vi "direct_ads_vol_T_pwpsatRho.vi"(5 "Density of adsorpt in kg/m3 (Input)":dbl, 7 "Saturation pressure in Pa (Input)":dbl, 8 "Error (Input)":errorcluster, 9 "Loading in kg/kg (Input)":dbl, 10 "Pressure in Pa (Input)":dbl, 11 "WorkingPair (Input)":T1={"no_iso"=1, "no_p_sat"=1, "path_db"="D:\\Driesel\\SorpLibLocal\\LabVIEW_wrapper\\data\\json\\sorpproplib_minimalExample.json", "wp_as"="silicagel", "wp_st"="123", "wp_iso"="DubininArctan1", "wp_rf"="water", "rf_rhol"="SaturatedLiquidDensity_EoS1", "no_rhol"=1, "rf_psat"="VaporPressure_EoS1"}) -> (0 "Error (Output)":errorcluster caption="Error(Output)", 3 "Equilibrium temperature in K (Output)":dbl)   [LabVIEW 2017]
doc: "direct_ads_vol_T_pwpsatRho:\n * ---------------------------\n *\n * Calculates equilibrium temperature T in K depending on equilibrium pressure\n * in Pa, equilibrium loading w in kg/kg, saturation pressure p_Sat in Pa and\n * density of adsorpt rho in kg/m³.\n *\n * Parameters:\n * -----------\n * double p_Pa:\n * Equilibrium pressure in Pa.\n * double w_kgkg:\n * Equilibrium loading in kg/kg.\n * double p_sat_Pa:\n * Saturation pressure in Pa.\n * double rho_kgm3:\n * Density of adsorpt in kg/m³.\n *\n * const char *path_db:\n * Path to database.\n * const char *wp_as:\n * Name of sorbent.\n * const char *wp_st:\n * Name of sub-type of sorbent.\n * const char *wp_rf:\n * Name of refrigerant.\n * const char *wp_iso:\n * Name of isotherm.\n * int no_iso:\n * ID of isotherm (i.e. when more than one isotherm is available)\n * const char *rf_psat:\n * Name of calculation approach for vapor pressure.\n * int no_p_sat:\n * ID of vapor pressure equation (i.e. when more than one equation is\n * available)\n * const char *rf_rhol:\n * Name of calculation approach for liquid density.\n * int no_rhol:\n * ID of liquid density equation (i.e. when more than one equation is\n * available)\n *\n * Returns:\n * --------\n * double:\n * Equilibrium temperature in K.\n *\n * Remarks:\n * --------\n * This function is only valid for isotherm models based on the volumetric\n * approach.\n * Uses internal equation of states to calculate vapor pressure, saturated\n * liquid density of adsorpt, derivative of vapor pressure wrt. temperature\n * and derivative of saturated liquid density of adsorpt wrt. temperature. If\n * equation of states are not implemented for refrigerant, function returns -1\n * and throws warning. If user want to use his own equation of states, this\n * function cannot be used and determination of root to calculate T must\n * be implemented by user.\n *\n * History:\n * --------\n * 07/07/2021, by Jannik Driesel (supervised by Mirko Engelpracht):\n * First implementation."
uses:
  data/win32bit/libsorpPropLib.dll
panel:
  # "Path to database"
  # "Name of sorbent"
  # "Name of sub-type of sorbent"
  # "Name of refrigerant"
  # "Name of isotherm"
  # "ID of isotherm"
  # "Name of calculation approach for vapor pressure"
  # "ID of vapor pressure equation"
  # "Name of calculation approach for liquid density"
  # "ID of liquid density equation"
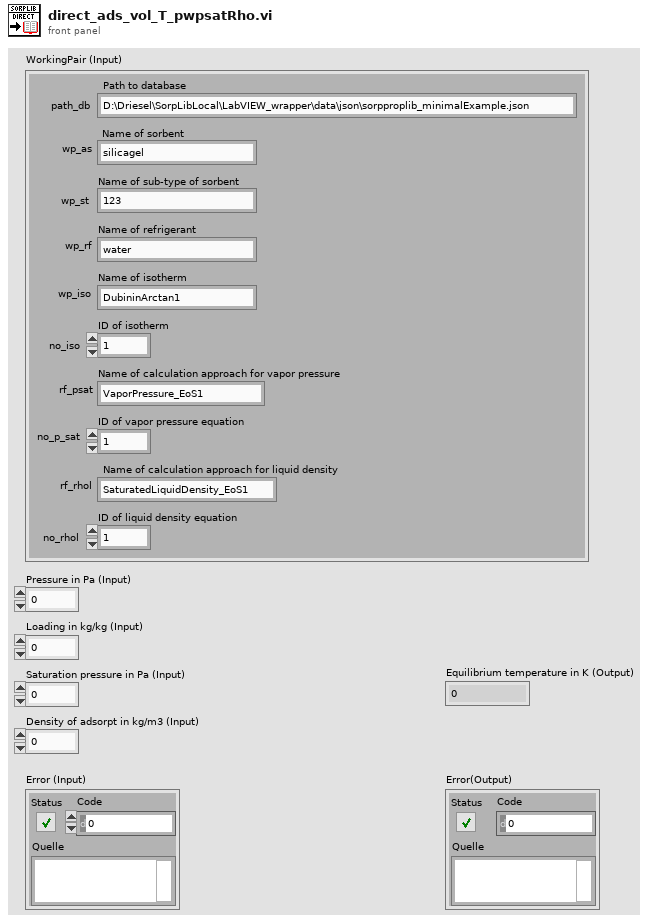
[diagram p1: front panel]
types:
  T1 = cluster{"no_iso":i32, "no_p_sat":i32, "path_db":string, "wp_as":string, "wp_st":string, "wp_iso":string, "wp_rf":string, "rf_rhol":string, "no_rhol":i32, "rf_psat":string}
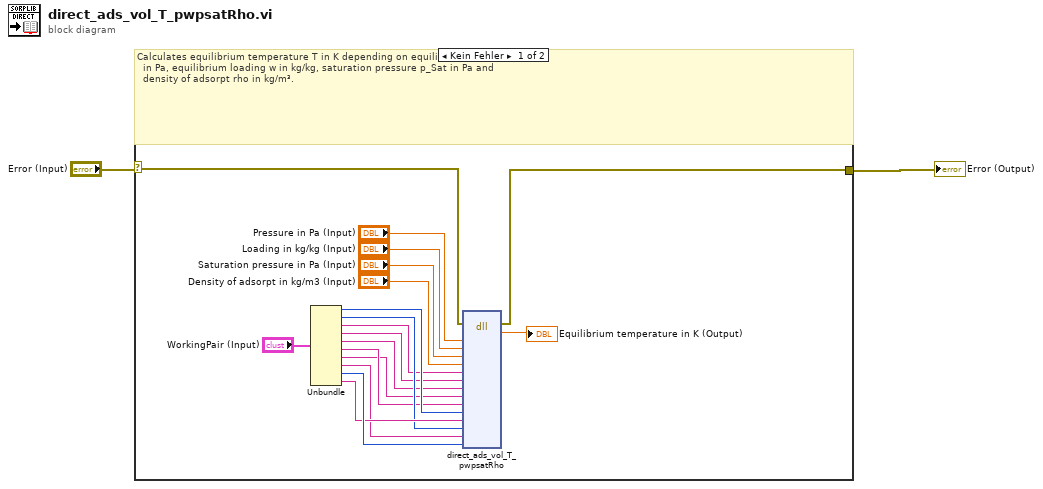
[diagram p0: block diagram]
diagram:
  n1 = case shown="Kein Fehler" "Error (Input)" {
    selector: "Error (Input)" -> [w8 w21]
    tunnel: [w7 w21] -> w1
    frame No Error {
      # "Calculates equilibrium temperature T in K depending on equilibrium pressure\n  in Pa, equilibrium loading w in kg/kg, saturation pressure p_Sat in Pa and\n  density of adsorpt rho in kg/m³."
      n2 = Unbundle("WorkingPair (Input)") -> ("no_iso"=w16:i32, "no_p_sat"=w17:i32, "path_db"=w10:string, "wp_as"=w11:string, "wp_st"=w12:string, "wp_iso"=w14:string, "wp_rf"=w13:string, "rf_rhol"=w15:string, "no_rhol"=w19:i32, "rf_psat"=w18:string)
      n3 = dll-call lib="D:/Driesel/SorpLibLocal/LabVIEW_wrapper/data/win32bit/libsorpPropLib.dll" fn="direct_ads_vol_T_pwpsatRho"(error in=w8, "p_Pa"="Pressure in Pa (Input)", "w_kgkg"="Loading in kg/kg (Input)", "p_sat_Pa"="Saturation pressure in Pa (Input)", "rho_kgm3"="Density of adsorpt in kg/m3 (Input)", "path_db"=w10, "wp_as"=w11, "wp_st"=w12, "wp_rf"=w13, "wp_iso"=w14, "no_iso"=w16, "rf_psat"=w18, "no_p_sat"=w17, "rf_rhol"=w15, "no_rhol"=w19) -> (error out=w7:errorcluster, "T_K"=→"Equilibrium temperature in K (Output)":dbl)  [unwired: 16 in, 1 out]
    }
    frame Error {
      # "Error - No calculations"
    }
  }
  "Error (Output)" <- w1
